vi "[RT] Cont Acq.vi"() -> ()   [LabVIEW 2015]
doc: "The continuous acquisition mode tells the FPGA to acquire points indefinitely until a stop command is issued or until an error is encountered (FIFO overflow, module underflow, and so on). \n\nIn this acquisition mode, explicitly call the appropriate rwfm_ConfigTiming VI and set the host application's data buffer to be many times larger than the read size. The examples use a 10X size by default. If the host application's data buffer fills, then the FPGA experiences a FIFO overflow causing the acquisition to stop."
uses:
  <vilib>/rvi/interface/nirviOpenFPGA/nirviOpenFPGA.xnode
  <vilib>/rvi/interface/nirviCloseFPGA/nirviCloseFPGA.xnode
  <vilib>/NI/cRIO Wfm/cRIO Wfm.lvlib
  <vilib>/NI/cRIO Wfm/AcqRead(Wfm).vi
  <vilib>/FPGAPlugInAG/cRIO-9074/niLvFpga_Open_cRIO-9074.vi
  <vilib>/rvi/interface/common/dynamic/niFpgaDynamicAddResources.vi
  <vilib>/FPGAPlugInAG/Dynamic/niLvFpga_Close_Dynamic.vi
  C:/Program Files (x86)/National Instruments/LabVIEW 2015/ProjectTemplates/Source/cRIOWfm/FPGA Bitfiles/DeltaSigMain_9074.lvbitx
  C:/Program Files (x86)/National Instruments/LabVIEW 2015/ProjectTemplates/Source/cRIOWfm/FPGA/[FPGA] DeltaSig Main.vi
  C:/Program Files (x86)/National Instruments/LabVIEW 2015/ProjectTemplates/Source/cRIOWfm/FPGA Bitfiles/SARAcqMain_9074.lvbitx
  C:/Program Files (x86)/National Instruments/LabVIEW 2015/ProjectTemplates/Source/cRIOWfm/FPGA/[FPGA] SAR Acq Main.vi
  <vilib>/NI/cRIO Wfm/ChannelConfig.ctl
panel:
  in  "Sample Rate":u32=51200
  in  "stop":bool
  out "Waveform Graph":waveform(sgl)[](graph)
  in  "Channel Info":T1=[{"Channel Name"="Mod1/ai0", "Sensitivity mV_EU"=1000.0, "EU"="V", "dB Ref EU"=1.0}, {"Channel Name"="Mod1/ai1", "Sensitivity mV_EU"=1000.0, "EU"="V", "dB Ref EU"=1.0}, {"Channel Name"="Mod1/ai2", "Sensitivity mV_EU"=1000.0, "EU"="V", "dB Ref EU"=1.0}, {"Channel Name"="Mod1/ai3", "Sensitivity mV_EU"=1000.0, "EU"="V", "dB Ref EU"=1.0}] caption="Channel Name      Scale [mV/EU]        EU           dB Ref [EU]" {"dB Ref EU" format="%#.2p"; "Sensitivity mV_EU" format="%.2f"}
  in  "Samps per Chan":i32=25600 caption="Samples per Channel"
  out "Buffer Backlog":dbl caption="RT Buffer Backlog [%]" format="%#.2g"
  # "Sampling Info"
  # "Channel Info"
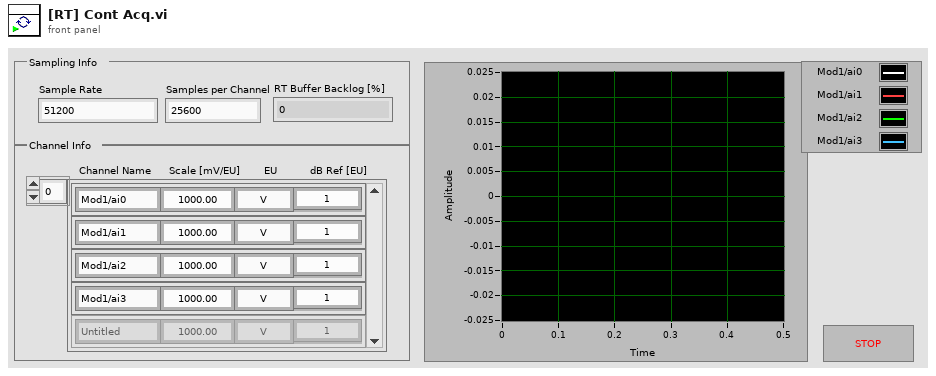
[diagram p1: front panel]
types:
  T1 = typedef "cRIO Wfm.lvlib/ChannelConfig.ctl" = cluster{"Channel Name":string, "Sensitivity mV_EU":dbl, "EU":string, "dB Ref EU":dbl}[]
  T2 = typedef "cRIO Wfm.lvlib/SamplingInfo.ctl" = cluster{"Number of Channels":i32, "Actual Samp Rate":dbl, "Chan Name Array":string[], "EU Chan Array":string[], "dB Ref Chan Array":dbl[]}
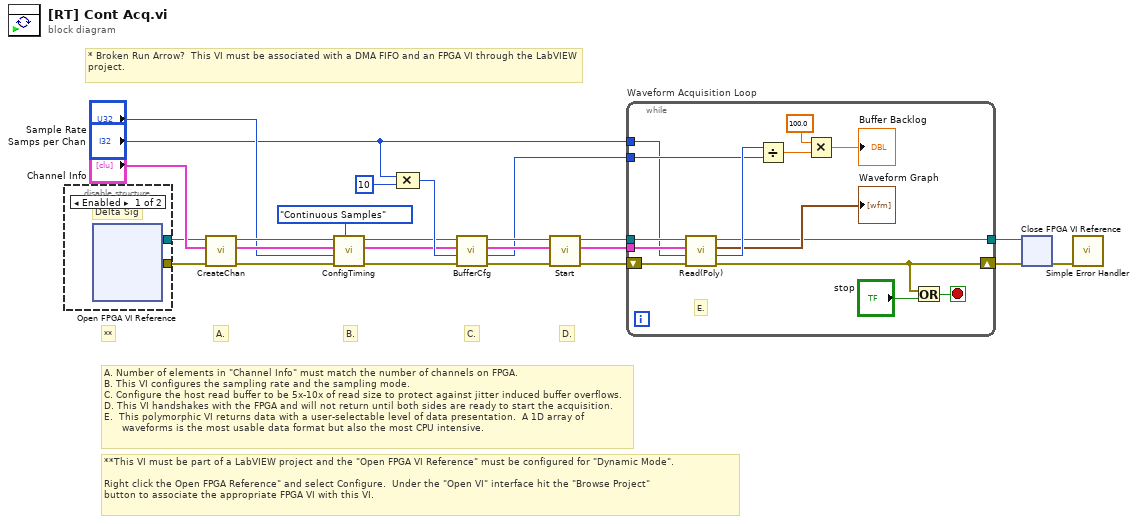
[diagram p0: block diagram]
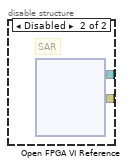
[diagram p2: hidden frame]
diagram:
  # "**This VI must be part of a LabVIEW project and the \"Open FPGA VI Reference\" must be configured for \"Dynamic Mode\".\n\nRight click the Open FPGA Reference\" and select Configure.  Under the \"Open VI\" interface hit the \"Browse Project\" \nbutton to associate the appropriate FPGA VI with this VI."
  # "* Broken Run Arrow?  This VI must be associated with a DMA FIFO and an FPGA VI through the LabVIEW project."
  # "A. Number of elements in \"Channel Info\" must match the number of channels on FPGA.\nB. This VI configures the sampling rate and the sampling mode.\nC. Configure the host read buffer to be 5x-10x of read size to protect against jitter induced buffer overflows.\nD. This VI handshakes with the FPGA and will not return until both sides are ready to start the acquisition.\nE.  This polymorphic VI returns data with a user-selectable level of data presentation.  A 1D array of     \n      waveforms is the most usable data format but also the most CPU intensive."
  # "**"
  # "D."
  # "C."
  # "B."
  # "A."
  n1 = disable-structure shown="Enabled" {
    disable-tunnel: [w26 w28] -> w2
    disable-tunnel: [w25 w27] -> w1
    frame Enabled {
      # "Delta Sig"
      n2 = xnode "Open FPGA VI Reference"() -> ("FPGA VI Reference Out"=w26:refnum<k20>, "error out"=w25:errorcluster)  [unwired: 2 in]
    }
    frame Disabled {
      # "SAR"
      n3 = xnode "Open FPGA VI Reference"() -> ("FPGA VI Reference Out"=w28:refnum<k20>, "error out"=w27:errorcluster)  [unwired: 2 in]
    }
  }
  n4 = call <vilib>:"CreateChan.vi"("error in"=w1, "Channel Info"="Channel Info", "Dynamic FPGA Ref"=w2) -> ("error out"=w6:errorcluster, "Sampling Info"=w10:T2, "Dynamic FPGA Ref Out"=w11:refnum<k20>)  [unwired: 1 in, 5 out]
  n5 = call <vilib>:"ConfigTiming.vi"("Sample Mode"=enum16{"Finite Samples", "Continuous Samples"}."Continuous Samples", "error in"=w6, "Sample Rate"="Sample Rate", "Sampling Info In"=w10, "Dynamic FPGA Ref"=w11) -> ("error out"=w7:errorcluster, "Sampling Info Out"=w8:T2, "Dynamic FPGA Ref Out"=w9:refnum<k20>)  [unwired: 3 in, 1 out]
  n6 = Compound Arithmetic op=MULTIPLY("Samps per Chan", 10 ("value")) -> (w16:i32)
  n7 = call <vilib>:"BufferCfg.vi"("error in"=w7, "Buffer Size [Samps per Chan]"=w16, "Sampling Info In"=w8, "Dynamic FPGA Ref"=w9) -> ("error out"=w17:errorcluster, "Buffer Size [Total Samples]"=w13:u32, "Sampling Info Out"=w15:T2, "Dynamic FPGA Ref Out"=w18:refnum<k20>)  [unwired: 4 out]
  n8 = call <vilib>:"Start.vi"("error in"=w17, "Sampling Info In"=w15, "Dynamic FPGA Ref"=w18) -> ("error out"=w23:errorcluster, "Sampling Info Out"=w14:T2, "Dynamic FPGA Ref Out"=w24:refnum<k20>)  [unwired: 6 out]
  n9 = while "Waveform Acquisition Loop" {
    tunnel: w24 -> [w35]
    tunnel: [w30] -> w22
    tunnel: w14 -> [w41]
    tunnel: w13 -> [w39]
    tunnel: "Samps per Chan" -> [w31]
    shift-right: [w29] -> w21
    shift-left: w23 -> [w42]
    stop <- w34 stop-if-true
    # "E."
    n10 = call-poly <vilib>:"Read(Poly).vi"("error in"=w42, "Samps Read per Chan"=w31, "Sampling Info"=w41, "Dynamic FPGA Ref"=w35) -> ("error out"=w29:errorcluster, "Samples Remaining"=w40:u32, "Wfm Data"=→"Waveform Graph":waveform(sgl)[], "Dynamic FPGA Ref Out"=w30:refnum<k20>)  [unwired: 2 in, 2 out]
    n11 = Divide(x=w40, y=w39) -> (x/y=w38:dbl)
    n12 = Multiply(x=100.0, y=w38) -> (x*y=→"Buffer Backlog":dbl)
    n13 = Or(x=w29, y="stop") -> (x .or. y?=w34:bool)
  }
  n14 = xnode "Close FPGA VI Reference"("FPGA VI Reference In"=w22, "error in"=w21) -> ("error out"=w19:errorcluster)
  n15 = call <vilib>:"Simple Error Handler.vi"("error in (no error)"=w19) -> ()  [unwired: 1 in, 8 out]
